vi "Validate Packet.vi"(8 "error in (no error)":errorcluster, 11 "ControlPacket in":refnum<class "ControlPacket.lvclass">) -> (0 "error out":errorcluster, 3 "ControlPacket out":refnum<class "ControlPacket.lvclass">)   [LabVIEW 2013, in "ControlPacket.lvclass"]
uses:
  ControlPacket.lvclass
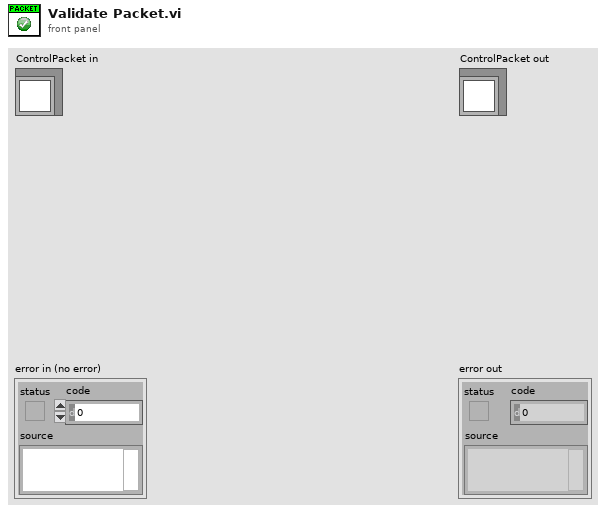
[diagram p1: front panel]
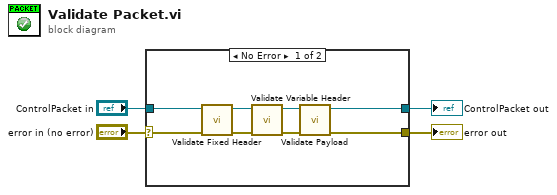
[diagram p0: block diagram]
diagram:
  n1 = case shown="No Error" "error in (no error)" {
    selector: "error in (no error)" -> [w6 w14]
    tunnel: [w5 w14] -> w3
    tunnel: [w7 w13] -> w1
    tunnel: "ControlPacket in" -> [w8 w13]
    frame No Error {
      n2 = call-dynamic "Validate Fixed Header.vi"("error in (no error)"=w6, "ControlPacket in"=w8) -> ("error out"=w11:errorcluster, "ControlPacket out"=w12:refnum<class "ControlPacket.lvclass">)  [unwired: 7 in, 1 out]
      n3 = call-dynamic "Validate Variable Header.vi"("error in (no error)"=w11, "ControlPacket in"=w12) -> ("error out"=w9:errorcluster, "ControlPacket out"=w10:refnum<class "ControlPacket.lvclass">)  [unwired: 7 in, 1 out]
      n4 = call-dynamic "Validate Payload.vi"("error in (no error)"=w9, "ControlPacket in"=w10) -> ("error out"=w5:errorcluster, "ControlPacket out"=w7:refnum<class "ControlPacket.lvclass">)  [unwired: 7 in, 1 out]
    }
    frame Error {
    }
  }
  "error out" <- w3
  "ControlPacket out" <- w1
